vi "Evaluate.vi"(0 "object in":refnum<class "OpenAngleToGoal.lvclass">, 1 "Game":refnum<class "Game.lvclass">, 2 "Point":dbl[](array[numeric]), 3 "Ally?":bool, 5 "error in (no error)":errorcluster) -> (14 "object out":refnum<class "OpenAngleToGoal.lvclass">, 16 "Evaluation":dbl, 19 "error out":errorcluster)   [LabVIEW 2023, in "OpenAngleToGoal.lvclass"]
uses:
  OpenAngleToGoal.lvclass
  Game_class/Game.lvclass
  Game_class/Game.lvclass/Game.ctl
  <vilib>/Analysis/_algsub.llb/Real Vector Norm.vi
  <vilib>/Analysis/baseanly.llb/Real Dot Product.vi
  Game_class/Read FieldRef.vi
  Field_class/Field.lvclass
  Utilities_class/Utilities.lvclass
  <vilib>/Analysis/NI_AALBase.lvlib
  <vilib>/Analysis/NI_AALPro.lvlib
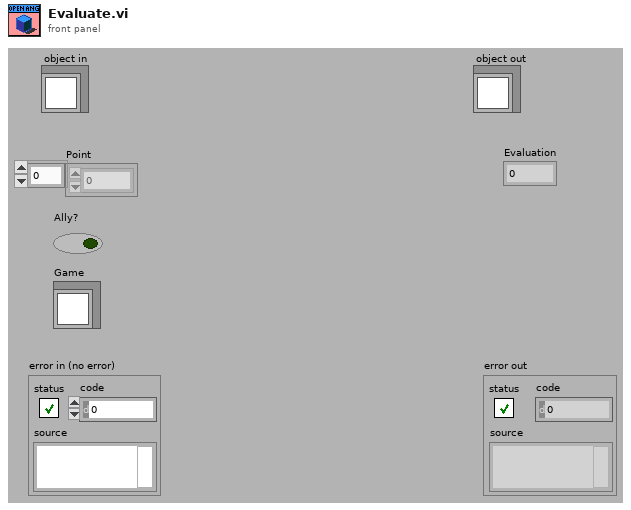
[diagram p1: front panel]
types:
  T1 = typedef "STPParameters.ctl" = cluster{"Skills":T2, "TestSkill":T4, "Events":cluster{"distanceToBallPossession":dbl, "timeForPossessionThreshold":dbl}, "Criteria":cluster{"OpenAngleToGoal":cluster{"minAngle":dbl, "maxAngle":dbl, "minEvaluation":dbl}, "PassDistance":cluster{"maxDistance":dbl, "minDistance":dbl}, "ShotTime":cluster{"shotSpeed":dbl, "keeperSpeed":dbl, "maxShotDistance":dbl}}, "MaxAngleToOneTouchShot":dbl}
  T2 = typedef "Skills.ctl" = cluster{"CirculateBall":T3, "ProtectBall":cluster{"DistanceFromBall":dbl}}
  T3 = typedef "CIrculateSkillParameters.ctl" = cluster{"rotationAngle":dbl, "velocityFactor":dbl, "OrientationFactor":dbl}
  T4 = typedef "TestSkills.ctl" = enum16{"AlignSkill", "PassSkill", "CirculateBall", "OneTouchShotSkill", "KickToSkill_v2", "ShootSkill", "InterceptBall", "GoToSkill_v2"}
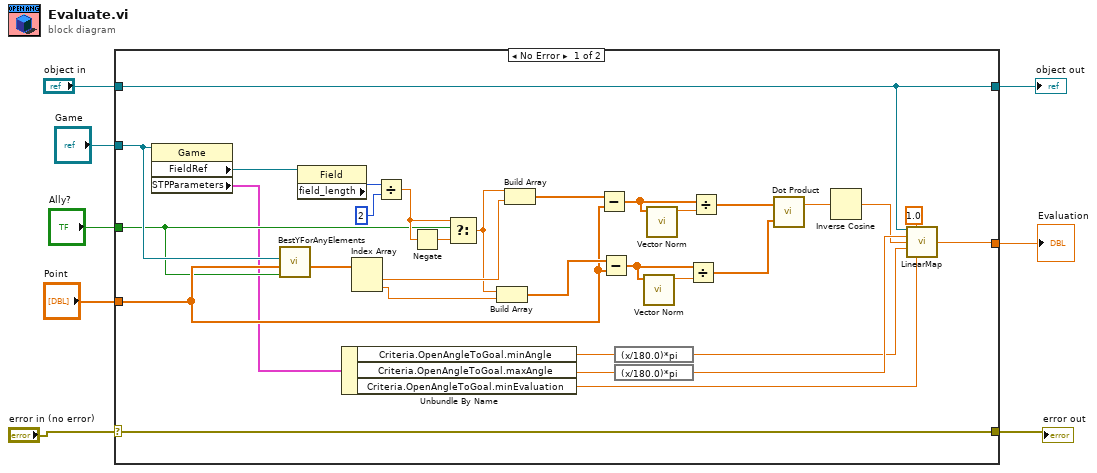
[diagram p0: block diagram]
diagram:
  n1 = case shown="No Error" "error in (no error)" {
    selector: "error in (no error)" -> [w40 w42]
    tunnel: "object in" -> [w13 w41]
    tunnel: [w40 w42] -> w6
    tunnel: [w13 w41] -> w5
    tunnel: "Game" -> [w24 _]
    tunnel: "Point" -> [w23 _]
    tunnel: "Ally?" -> [w19 _]
    tunnel: [w9 _] -> w1
    frame No Error {
      n2 = property class="Game"(reference=w24) -> ("FieldRef"=w36:refnum<class "Field.lvclass">, "STPParameters"=w18:T1)  [unwired: 1 in, 2 out]
      n3 = call "BestYForAnyElements.vi"("inimigos"=w19, "Position to be analyzed"=w23, "Game"=w24) -> ("Gap Coord"=w39:dbl[])  [unwired: 5 in, 3 out]
      n4 = property class="Field"(reference=w36) -> ("field_length"=w35:i32)  [unwired: 1 in, 2 out]
      n5 = Unbundle By Name(w18) -> ("Criteria.OpenAngleToGoal.minAngle"=w16:dbl, "Criteria.OpenAngleToGoal.maxAngle"=w17:dbl, "Criteria.OpenAngleToGoal.minEvaluation"=w14:dbl)
      n6 = Index Array(array=w39) -> (element #1=w38:dbl, element #2=w37:dbl)  [unwired: 2 in]
      n7 = Divide(x=w35, y=2) -> (x/y=w20:dbl)
      n8 = Negate(x=w20) -> (-x=w21:dbl)
      n9 = Select(t=w20, s=w19, f=w21) -> (s? t:f=w22:dbl)
      n10 = Build Array(w22, w37) -> (w32:dbl[])
      n11 = Build Array(w22, w38) -> (w33:dbl[])
      n12 = Subtract(x=w33, y=w23) -> (x-y=w30:dbl[])
      n13 = Subtract(x=w32, y=w23) -> (x-y=w27:dbl[])
      n14 = expression code="(x/180.0)*pi" ("degrees to radians")(w16) -> (w10:dbl)
      n15 = expression code="(x/180.0)*pi" ("degrees to radians")(w17) -> (w12:dbl)
      n16 = call-poly <vilib>:"Vector Norm.vi"("Input Vector"=w27) -> ("norm"=w28:dbl)  [unwired: 9 in, 1 out]
      n17 = call-poly <vilib>:"Vector Norm.vi"("Input Vector"=w30) -> ("norm"=w29:dbl)  [unwired: 9 in, 1 out]
      n18 = Divide(x=w27, y=w28) -> (x/y=w25:dbl[])
      n19 = Divide(x=w30, y=w29) -> (x/y=w26:dbl[])
      n20 = call-poly <vilib>:"Dot Product.vi"("Y Vector"=w25, "X Vector"=w26) -> ("X * Y"=w31:dbl)  [unwired: 1 out]
      n21 = Inverse Cosine(1:w31) -> (0:w11:dbl)
      n22 = call-dynamic "LinearMap.vi"("Criterion in"=w13, "MaxEvalutation"=1.0, "MaxVal"=w12, "Val"=w11, "MinVal"=w10, "MinEvaluation"=w14) -> ("Evaluation"=w9:dbl)  [unwired: 7 in, 2 out]
    }
    frame Error {
    }
  }
  "error out" <- w6
  "object out" <- w5
  "Evaluation" <- w1
